vi "APC_ReplaceInNames.vi"(1 "string":string[](array[string])) -> (0 "result string":string[](array[string]))   [LabVIEW 2020]
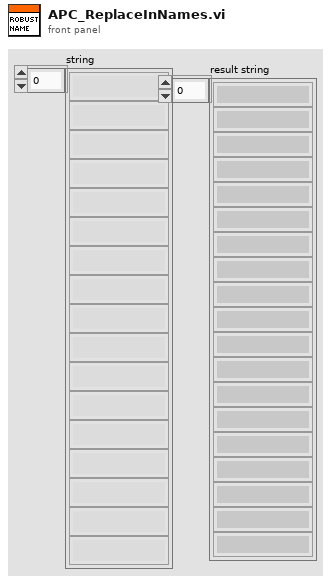
[diagram p1: front panel]
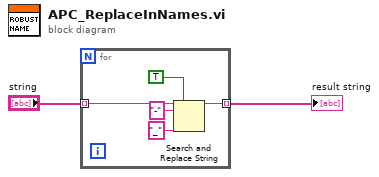
[diagram p0: block diagram]
diagram:
  n1 = for {
    tunnel: "string" -> [w7] mode=indexing
    tunnel: [w4] -> w1 mode=indexing
    n2 = Search and Replace String(replace all?=TRUE ("replace all? (F)"), input string=w7, search string="-", replace string="_" ("replace string (\"\")")) -> (result string=w4:string)  [unwired: 4 in, 3 out]
  }
  "result string" <- w1
